vi "Set Cursors.vi"(8 "Error In":errorcluster, 9 "Interval [s]":dbl=0.0001 min=1e-06 max=0.0001 step=1e-06 format="%#_6p", 10 "Start [s]":dbl[](array[numeric]) format="%#_6p", 11 "Waveform Graph":refnum<vi>) -> (0 "error out":errorcluster)   [LabVIEW 2019]
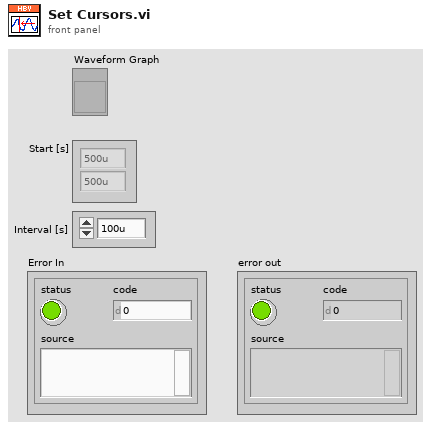
[diagram p1: front panel]
types:
  T1 = typedef "LVCursorListTypeDef.ctl" = cluster{"Name":string, "Color":u32, "Style":u8, "Point Style":u8, "Name Visible":bool, "Allow Drag":bool, "Cursor Mode":u32, "Plot":i32, "Index":i32, "Position":cluster{"X":dbl, "Y":dbl}, "X Scale":u32, "Y Scale":u32, "Watch Plots":i32[], "Watch All Plots":bool, "Plot Area":i32, "Label Offset":cluster{"X":dbl, "Y":dbl}}[]
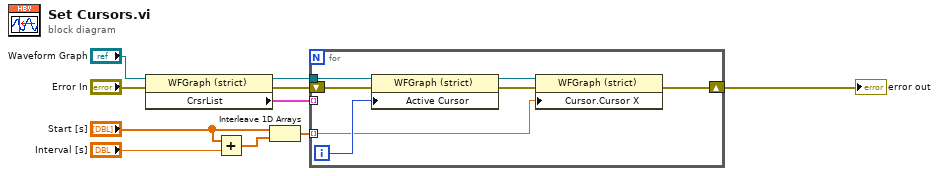
[diagram p0: block diagram]
diagram:
  n1 = property class="WFGraph (strict)"(reference="Waveform Graph", error in="Error In") -> (reference out=w5:refnum<vi>, error out=w7:errorcluster, "CrsrList"=w6:T1)
  n2 = Add(x="Start [s]", y="Interval [s]") -> (x+y=w2:dbl[])
  n3 = Interleave 1D Arrays("Start [s]", w2) -> (w1:dbl[])
  n4 = for {
    tunnel: w6 -> [_] mode=indexing
    tunnel: w5 -> [w17]
    shift-right: [w13] -> w10
    shift-left: w7 -> [w15]
    tunnel: w1 -> [w12] mode=indexing
    i -> [w16]
    n5 = property class="WFGraph (strict)"(reference=w17, error in=w15, "Active Cursor"=w16) -> (reference out=w11:refnum<vi>, error out=w14:errorcluster)
    n6 = property class="WFGraph (strict)"(reference=w11, error in=w14, "Cursor.Cursor X"=w12) -> (error out=w13:errorcluster)  [unwired: 1 out]
  }
  "error out" <- w10
